vi "Robot Global Data.vi"() -> ()   [LabVIEW 2015]
doc: "This global VI can contain as many global variables as you need. Place a control on the panel, give it a good name. To read or write to it from a VI, drag the icon to the diagram of that VI. You can also drag from the project. Click on the node to change which global you access. You shouldn't have multiple locations writing to a global or it will cause a race-condition."
uses:
  <vilib>/Rock Robotics/WPI/Camera/WPI_CameraImageSize.ctl
  <vilib>/Rock Robotics/WPI/DriverStation/WPI_DriverStationRobotMode2.ctl
  ArmStates.ctl
panel:
  out "Teleop First call":bool
  out "Arm Hold Cylinder":bool
  out "Pto break on":bool=TRUE
  out "Pto on":bool
  out "Left Drive Overide":dbl
  out "Right Drive Overide":dbl
  out "Overide Drives":bool
  out "Spin Up Wheels From Auton":bool
  out "Shoot From Auton":bool
  out "Shooting Done":bool
  in  "Desired Arm State From Auton":T1
  in  "Arm State":T1
  out "Arm Power Vbus":bool
  out "Roller":bool
  out "Desired Arm Position":dbl
  out "Vision Distance From Target":dbl
  out "Shooter Speed Mode":bool
  out "Porticullis position":dbl
  out "Drive Positon":dbl
  out "Drawbridge Position":dbl
  out "Sally Door Position":dbl
  out "Arm hic up Position":dbl
  out "Arm up Position":dbl
  out "Arm down Position":dbl
  out "Arm base offset":dbl
  out "Current Arm Case":dbl
  out "Arm Control Method":dbl
  out "Back Finger":bool
  out "Front Finger":bool
  out "Shooter Speed":dbl
  out "Roller speed":dbl
  out "Arm output":dbl
  out "Vision Target Right Bound":dbl
  out "Vision Target Left Bound":dbl
  in  "Robot Mode":T2
  out "ms to process":u32
  in  "image size":T3=enum."320x240"
  in  "Enable Vision":bool
  # "Arm control"
  # "Shooter control"
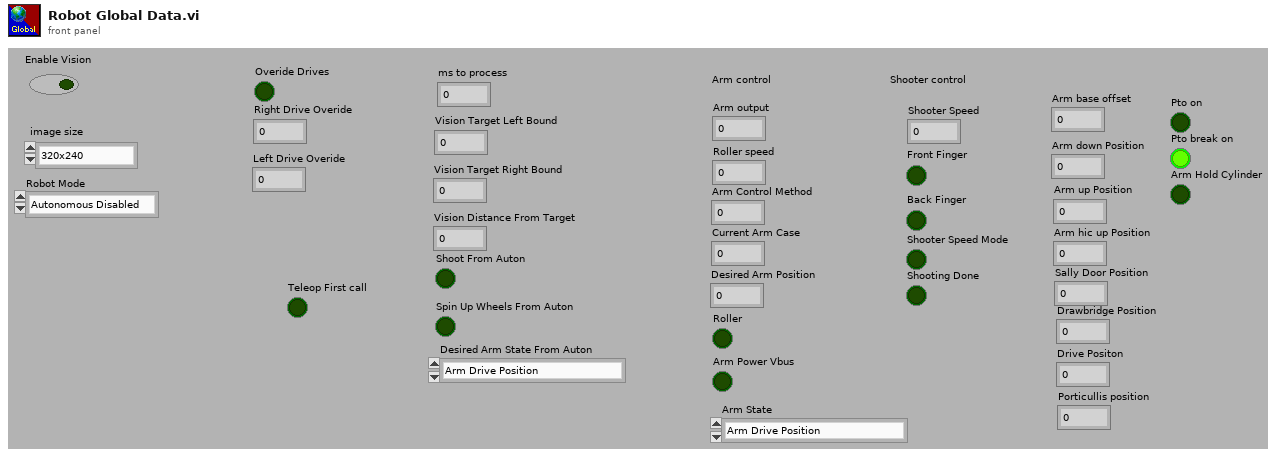
[diagram p1: front panel]
types:
  T1 = typedef "ArmStates.ctl" = enum16{"Arm Drive Position", "Winch Up", "Level Arm", "Hold Climb", "Drawbridge Drive Forward", "Shoot Position", "Roll Out", "Hic Up Rollers Off", "Draw Bridge Arm Down", "Harvest Back Down", "Harvest Hic up", "Portcullis", "Sally Door", "Harvest", "Arm Up", "Arm Down"}
  T2 = typedef "WPI_DriverStationRobotMode2.ctl" = enum16{"Autonomous Disabled", "Autonomous Enabled", "Teleop Disabled", "Teleop Enabled", "Disconnected", "Finish", "Test Disabled", "Test Enabled", "Emergency Stopped"}
  T3 = typedef "WPI_CameraImageSize.ctl" = enum16{"640x480", "320x240", "160x120", "Custom"}
diagram:
